vi "getHostname.vi"(8 "error in":errorcluster, 11 "connection ID":refnum<k5>) -> (0 "error out":errorcluster, 2 "available":string, 3 "connection ID":refnum<k5>)   [LabVIEW 2016]
doc: "Return device hostname"
panel:
  out "params_cluster":cluster{"Numeric":i32}
  in  "Params_cluster":cluster{"Numeric":dbl}
  in  "results_cluster":cluster{"errNo":i32, "available":string}
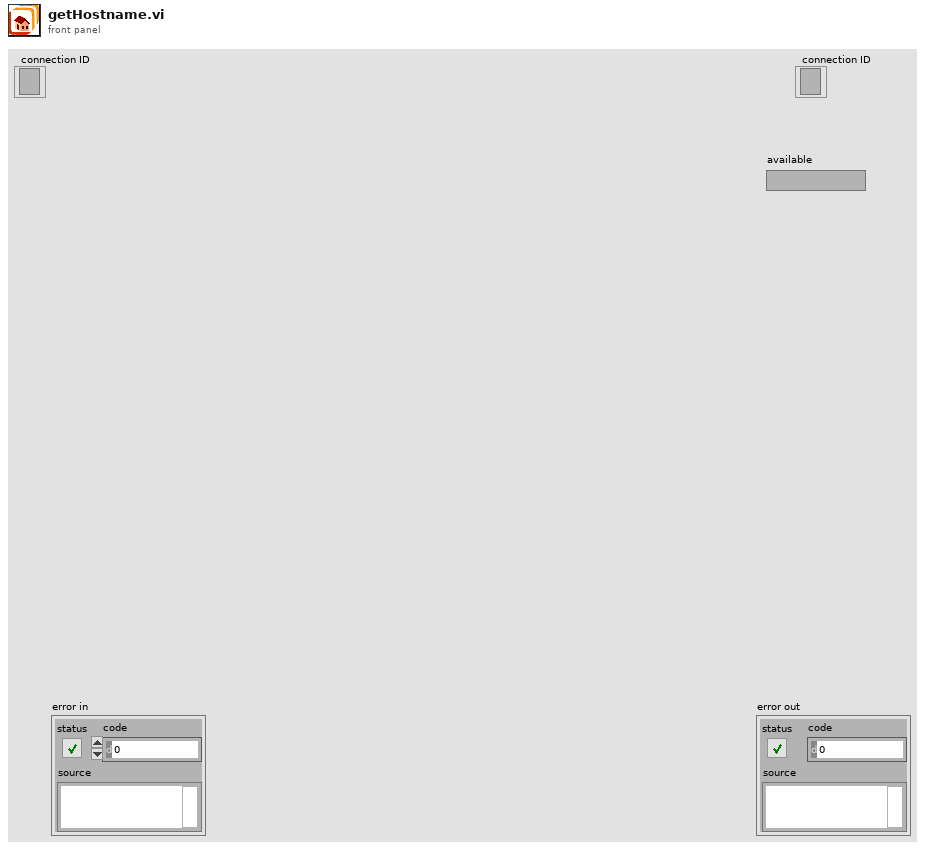
[diagram p1: front panel]
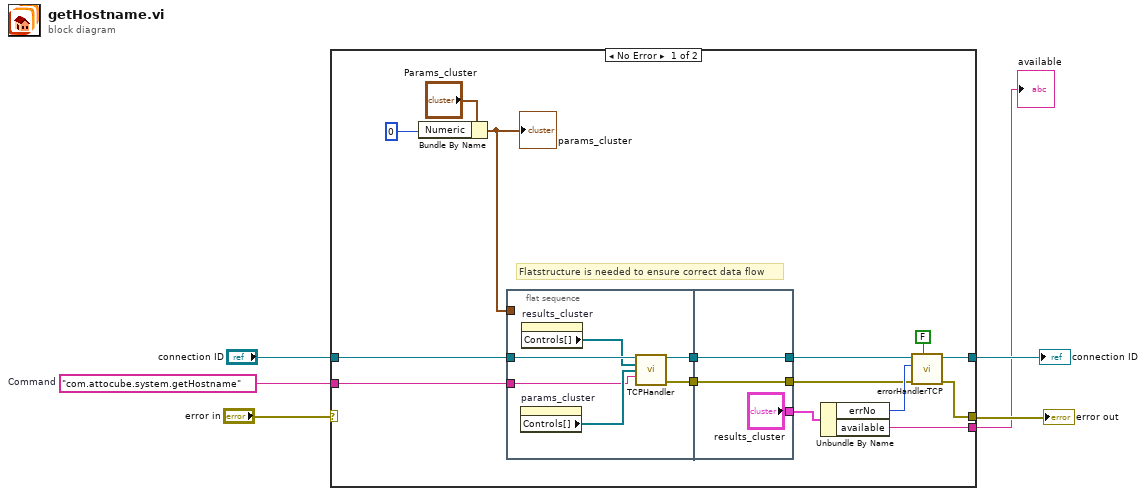
[diagram p0: block diagram]
diagram:
  w2 = "com.attocube.system.getHostname"  # Command
  n1 = case shown="No Error" "error in" {
    selector: "error in" -> [_ w32]
    tunnel: [w19 w32] -> w6
    tunnel: [w21 w31] -> w5
    tunnel: "connection ID" -> [w18 w31]
    tunnel: w2 -> [w12 _]
    tunnel: [w7 _] -> w1
    frame No Error {
      # "Flatstructure is needed to ensure correct data flow"
      n2 = Bundle By Name(cluster="Params_cluster", "Numeric"=0) -> (w9:cluster{"Numeric":dbl})
      "params_cluster" <- w9
      n3 = flat-sequence {
        tunnel: [w26] -> w14
        tunnel: w18 -> [w27]
        tunnel: w12 -> [w23]
        tunnel: [w22] -> w10
        tunnel: w9 -> [_]
        tunnel: ["results_cluster"] -> w15
        tunnel: [w30] -> w17
        tunnel: w14 -> [w30]
        tunnel: [w28] -> w11
        tunnel: w10 -> [w28]
        frame #0 {
          n4 = property on="params_cluster" class="Clust (strict)"() -> ("Controls[]"=w24:refnum<vi>[])  [unwired: 2 in, 2 out]
          n5 = property on="results_cluster" class="Clust (strict)"() -> ("Controls[]"=w25:refnum<vi>[])  [unwired: 2 in, 2 out]
          n6 = call "TCPHandler.vi"("connection ID"=w27, "results_cluster"=w25, "params_cluster"=w24, "method"=w23) -> ("connection ID"=w26:refnum<k5>, "error"=w22:errorcluster)  [unwired: 8 in, 2 out]
        }
        frame #1 {
        }
      }
      n7 = Unbundle By Name(w15) -> ("errNo"=w16:i32, "available"=w7:string)
      n8 = call "errorHandlerTCP.vi"("show popup"=FALSE, "error in"=w11, "error number"=w16, "connection ID"=w17) -> ("error out"=w19:errorcluster, "connection ID"=w21:refnum<k5>)  [unwired: 6 in]
    }
    frame Error {
    }
  }
  "error out" <- w6
  "connection ID" <- w5
  "available" <- w1
